vi "Results Analyser.vi"() -> ()   [LabVIEW 2020]
panel:
  in  "Reset":bool
  out "Total Files":u32
  in  "Calculate":bool
  in  "Quit":bool
  in  "Lower Limit":string
  in  "Upper Limit":string
  out "Analysis":T1={"Target"=4.0, "Average"=4.07375, "Standard Deviation"=0.10336309095334055, "Cp"=3.2248777610937, "Cpu"=2.9870430262130383, "Cpl"=3.462712495974362, "Cpk"=2.9870430262130383}
  out "Results":dbl[](array[numeric])=[4.0, 4.1, 4.07, 4.1, 4.0, 4.05, 4.3, 3.97]
  out "Graph":picture
  out "Histogram":picture
  in  "Tests":i32(listbox)
  out "Test List":string[](array[string])
  out "Files":path[](array[path])
  in  "Add Files":bool
  in  "Aborted":bool
  in  "Fail":bool
  in  "Pass":bool=TRUE
  in  "Results Directory":path=path "C:/Results/test"
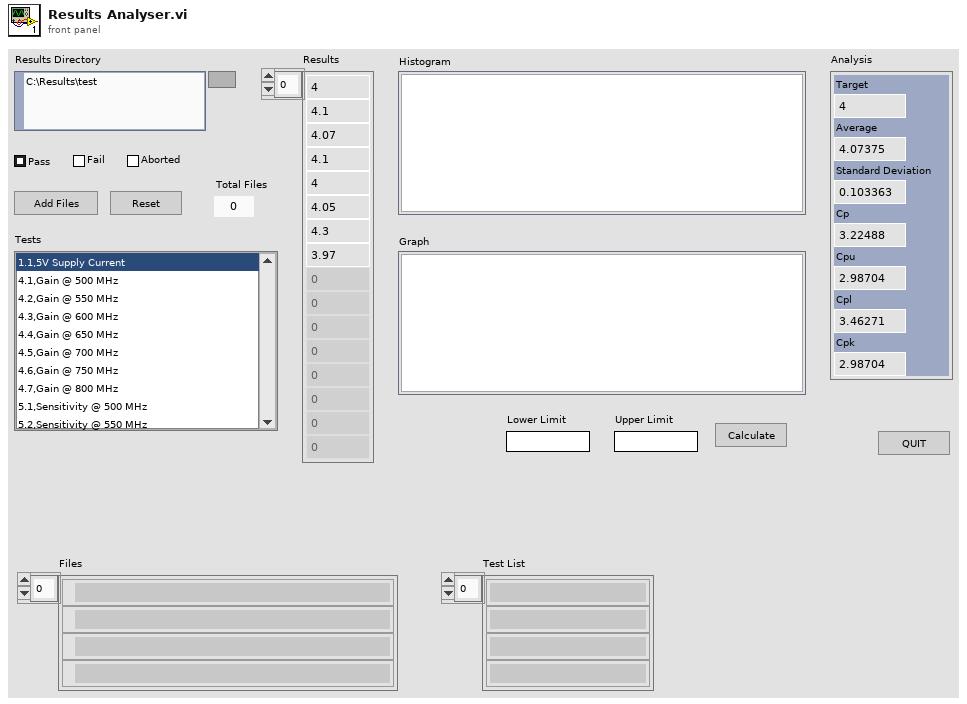
[diagram p1: front panel]
types:
  T1 = cluster{"Target":dbl, "Average":dbl, "Standard Deviation":dbl, "Cp":dbl, "Cpu":dbl, "Cpl":dbl, "Cpk":dbl}
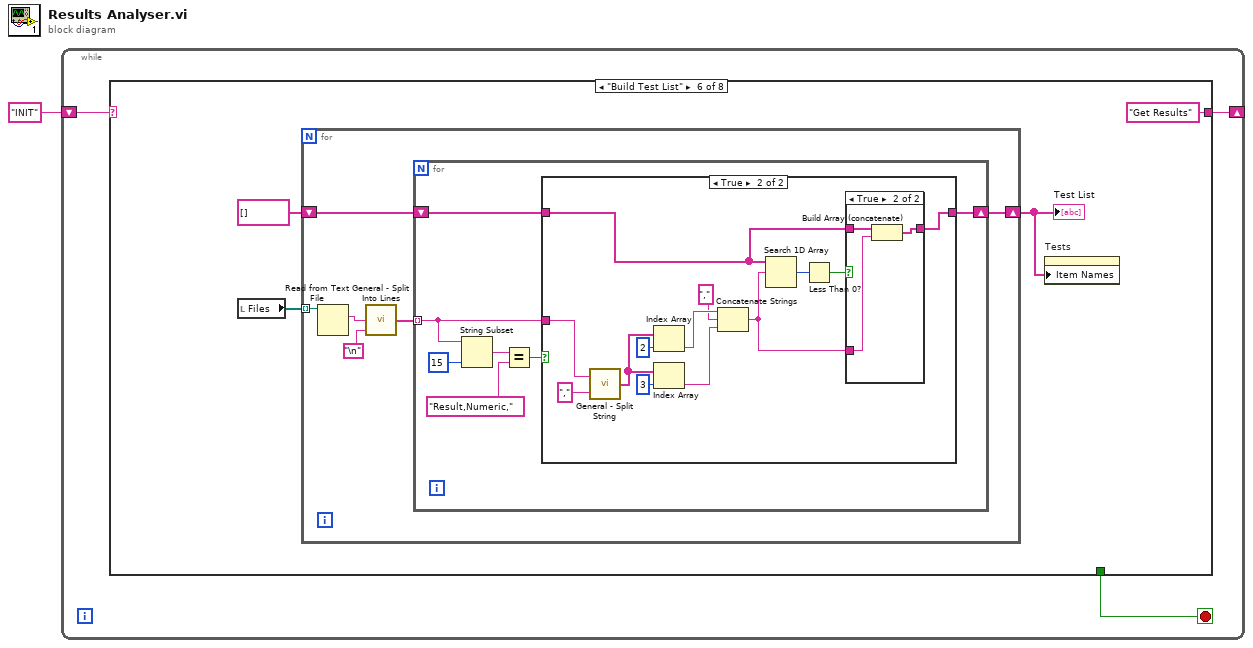
[diagram p0: block diagram]
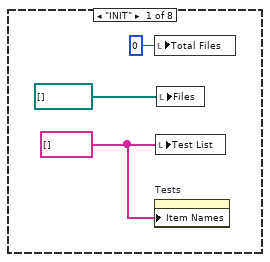
[diagram p2: hidden frame]
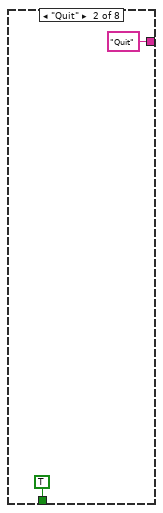
[diagram p3: hidden frame]
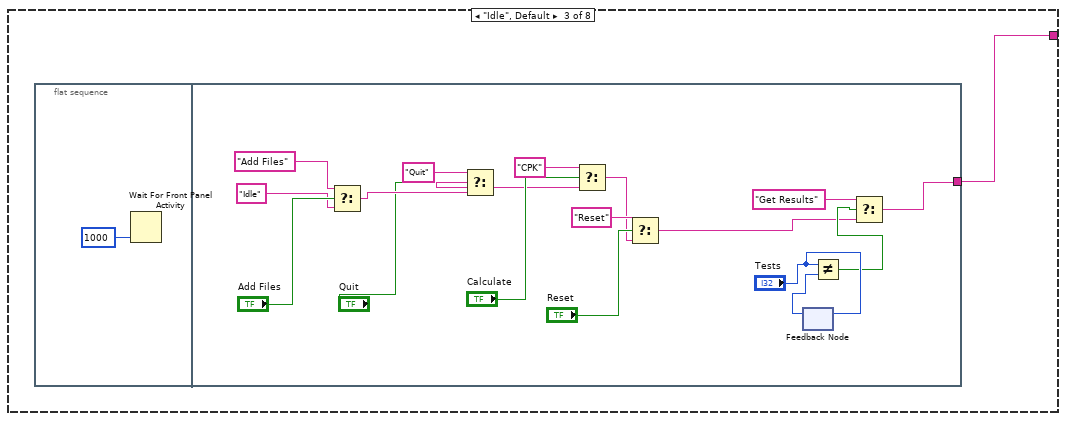
[diagram p4: hidden frame]
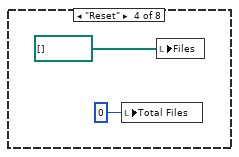
[diagram p5: hidden frame]
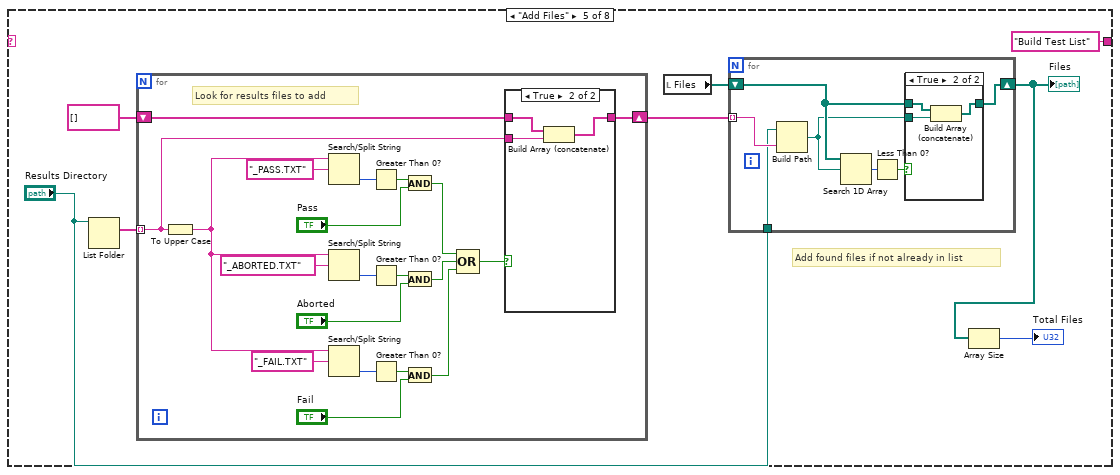
[diagram p6: hidden frame]
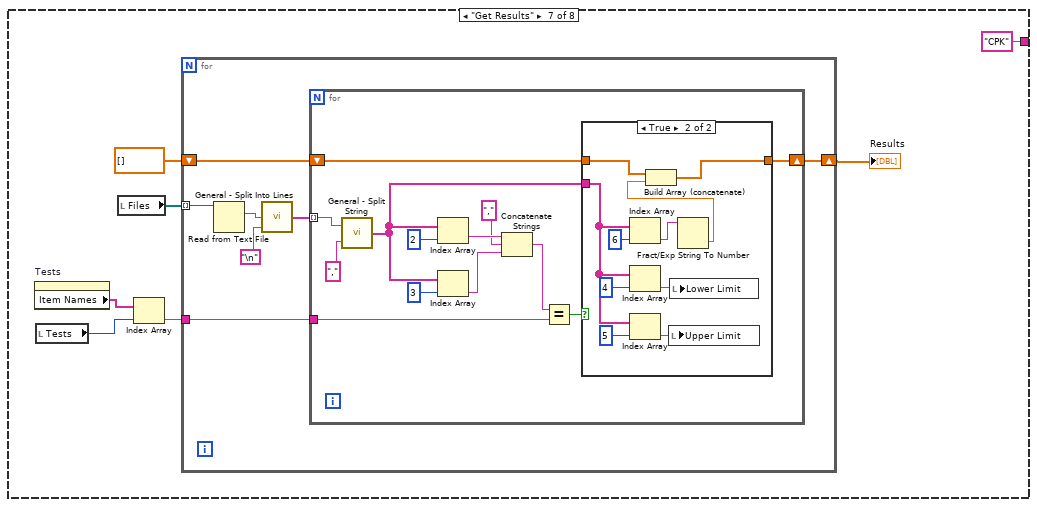
[diagram p11: hidden frame]
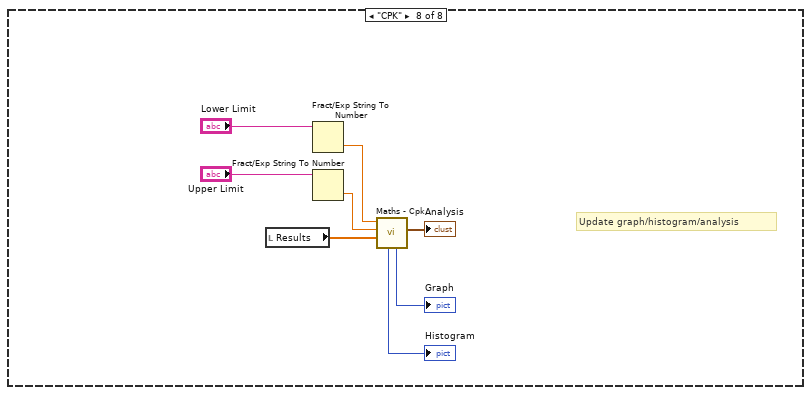
[diagram p13: hidden frame]
diagram:
  n1 = while {
    shift-right: [w3] -> _
    shift-left: "INIT" -> [w4]
    stop <- w2 stop-if-true
    n2 = case shown="\"Build Test List\"" w4 {
      tunnel: [_ "Quit" w10 _ "Build Test List" "Get Results" "CPK" _] -> w3
      tunnel: [_ TRUE _ _ _ _ _ _] -> w2
      frame "INIT" {
        w5 = string[] []
        n3 = local write "Total Files"(u32 0 ("Total Files")) -> ()
        n4 = property on="Tests" class="LstBox (strict)"("Item Names"=w5) -> ()  [unwired: 2 in, 2 out]
        n5 = local write "Test List"(w5) -> ()
        n6 = local write "Files"(path[] []) -> ()
      }
      frame "Quit" {
      }
      frame "Idle", Default {
        n7 = flat-sequence {
          tunnel: [w20] -> w10
          frame #0 {
            n8 = Wait For Front Panel Activity(1:1000 ("timeout ms (-1 never timeout)")) -> ()  [unwired: 2 in, 1 out]
          }
          frame #1 {
            n9 = Select(t="Add Files", s="Add Files", f="Idle") -> (s? t:f=w25:string)
            n10 = Select(t="Quit", s="Quit", f=w25) -> (s? t:f=w24:string)
            n11 = Select(t="CPK", s="Calculate", f=w24) -> (s? t:f=w13:string)
            n12 = Select(t="Reset", s="Reset", f=w13) -> (s? t:f=w12:string)
            n13 = feedback-in #1("Tests") -> ()
            n14 = feedback #1() -> (w18:i32)  [unwired: 1 in]
            n15 = Not Equal?(x="Tests", y=w18) -> (x != y?=w16:bool)
            n16 = Select(t="Get Results", s=w16, f=w12) -> (s? t:f=w20:string)
          }
        }
      }
      frame "Reset" {
        n17 = local write "Total Files"(u32 0 ("Total Files")) -> ()
        n18 = local write "Files"(path[] []) -> ()
      }
      frame "Add Files" {
        # "Add found files if not already in list"
        n19 = List Folder(path="Results Directory") -> (filenames=w39:string[])  [unwired: 3 in, 3 out]
        n20 = for {
          tunnel: w39 -> [w51] mode=indexing
          shift-right: [w53] -> w37
          shift-left: string[] [] -> [w54]
          # "Look for results files to add"
          n21 = To Upper Case(1:w51) -> (0:w52:string)
          n22 = Search/Split String(string=w52, search string/char (-)="_PASS.TXT") -> (offset of match=w64:i32)  [unwired: 1 in, 2 out]
          n23 = Search/Split String(string=w52, search string/char (-)="_ABORTED.TXT") -> (offset of match=w63:i32)  [unwired: 1 in, 2 out]
          n24 = Search/Split String(string=w52, search string/char (-)="_FAIL.TXT") -> (offset of match=w62:i32)  [unwired: 1 in, 2 out]
          n25 = Greater Than 0?(x=w64) -> (x > 0?=w61:bool)
          n26 = Greater Than 0?(x=w63) -> (x > 0?=w60:bool)
          n27 = Greater Than 0?(x=w62) -> (x > 0?=w59:bool)
          n28 = And(x=w61, y="Pass") -> (x .and. y?=w67:bool)
          n29 = And(x=w60, y="Aborted") -> (x .and. y?=w66:bool)
          n30 = And(x=w59, y="Fail") -> (x .and. y?=w65:bool)
          n31 = Compound Arithmetic op=OR(w67, w66, w65) -> (w55:bool)
          n32 = case shown="True" w55 {
            tunnel: w54 -> [w71 w73]
            tunnel: [w71 w74] -> w53
            tunnel: w51 -> [_ w72]
            frame False {
            }
            frame True {
              n33 = Build Array (concatenate)(w73, w72) -> (w74:string[])
            }
          }
        }
        n34 = local read "Files"() -> (w33:path[])
        n35 = for {
          tunnel: w37 -> [w46] mode=indexing
          tunnel: "Results Directory" -> [w45]
          shift-right: [w40] -> w32
          shift-left: w33 -> [w42]
          n36 = Build Path(base path=w45, name or relative path=w46) -> (appended path=w41:path)
          n37 = Search 1D Array(1D array=w42, element=w41) -> (index of element=w44:i32)  [unwired: 1 in]
          n38 = Less Than 0?(x=w44) -> (x < 0?=w43:bool)
          n39 = case shown="True" w43 {
            tunnel: w42 -> [w47 w50]
            tunnel: [w47 w49] -> w40
            tunnel: w41 -> [_ w48]
            frame False {
            }
            frame True {
              n40 = Build Array (concatenate)(w50, w48) -> (w49:path[])
            }
          }
        }
        "Files" <- w32
        n41 = Array Size(array=w32) -> (size(s)=→"Total Files":i32)
      }
      frame "Build Test List" {
        n42 = local read "Files"() -> (w78:path[])
        n43 = for {
          tunnel: w78 -> [w84] mode=indexing
          shift-right: [w79] -> w76
          shift-left: string[] [] -> [w80]
          n44 = Read from Text File(file (use dialog)=w84) -> (text=w83:string)  [unwired: 3 in, 3 out]
          n45 = call "General - Split Into Lines.vi"("Line Termination Character"="\n", "String"=w83) -> ("Array"=w81:string[])  [unwired: 3 in]
          n46 = for {
            tunnel: w81 -> [w87] mode=indexing
            shift-right: [w85] -> w79
            shift-left: w80 -> [w86]
            n47 = String Subset(string=w87, length (rest)=15 ("length (rest)")) -> (substring=w90:string)  [unwired: 1 in]
            n48 = Equal?(x=w90, y="Result,Numeric,") -> (x = y?=w88:bool)
            n49 = case shown="True" w88 {
              tunnel: w87 -> [_ w105]
              tunnel: w86 -> [w92 w95]
              tunnel: [w92 w94] -> w85
              frame False {
              }
              frame True {
                n50 = call "General - Split String.vi"("Delimeter (;)"=",", "String"=w105) -> ("String Array"=w103:string[])
                n51 = Index Array(array=w103, index=2) -> (element=w100:string)
                n52 = Index Array(array=w103, index=3) -> (element=w99:string)
                n53 = Concatenate Strings(w100, ",", w99) -> (w93:string)
                n54 = Search 1D Array(1D array=w95, element=w93) -> (index of element=w97:i32)  [unwired: 1 in]
                n55 = Less Than 0?(x=w97) -> (x < 0?=w96:bool)
                n56 = case shown="True" w96 {
                  tunnel: w95 -> [w106 w109]
                  tunnel: [w106 w108] -> w94
                  tunnel: w93 -> [_ w107]
                  frame False {
                  }
                  frame True {
                    n57 = Build Array (concatenate)(w109, w107) -> (w108:string[])
                  }
                }
              }
            }
          }
        }
        "Test List" <- w76
        n58 = property on="Tests" class="LstBox (strict)"("Item Names"=w76) -> ()  [unwired: 2 in, 2 out]
      }
      frame "Get Results" {
        n59 = property on="Tests" class="LstBox (strict)"() -> ("Item Names"=w116:string[])  [unwired: 2 in, 2 out]
        n60 = local read "Tests"() -> (w115:i32)
        n61 = local read "Files"() -> (w113:path[])
        n62 = Index Array(array=w116, index=w115) -> (element=w114:string)
        n63 = for {
          tunnel: w114 -> [w119]
          tunnel: w113 -> [w123] mode=indexing
          shift-right: [w117] -> w112
          shift-left: dbl[] [] -> [w118]
          n64 = Read from Text File(file (use dialog)=w123) -> (text=w122:string)  [unwired: 3 in, 3 out]
          n65 = call "General - Split Into Lines.vi"("Line Termination Character"="\n", "String"=w122) -> ("Array"=w120:string[])  [unwired: 3 in]
          n66 = for {
            tunnel: w120 -> [w136] mode=indexing
            tunnel: w119 -> [w128]
            shift-right: [w126] -> w117
            shift-left: w118 -> [w127]
            n67 = call "General - Split String.vi"("Delimeter (;)"=",", "String"=w136) -> ("String Array"=w125:string[])
            n68 = Index Array(array=w125, index=2) -> (element=w132:string)
            n69 = Index Array(array=w125, index=3) -> (element=w131:string)
            n70 = Concatenate Strings(w132, ",", w131) -> (w129:string)
            n71 = Equal?(x=w129, y=w128) -> (x = y?=w124:bool)
            n72 = case shown="True" w124 {
              tunnel: w127 -> [w137 w147]
              tunnel: [w137 w146] -> w126
              tunnel: w125 -> [_ w142]
              frame False {
              }
              frame True {
                n73 = Index Array(array=w142, index=6) -> (element=w144:string)
                n74 = Index Array(array=w142, index=4) -> (element=w139:string)
                n75 = Index Array(array=w142, index=5) -> (element=w138:string)
                n76 = local write "Upper Limit"(w138) -> ()
                n77 = local write "Lower Limit"(w139) -> ()
                n78 = Fract/Exp String To Number(string=w144) -> (number=w143:dbl)  [unwired: 3 in, 1 out]
                n79 = Build Array (concatenate)(w147, w143) -> (w146:dbl[])
              }
            }
          }
        }
        "Results" <- w112
      }
      frame "CPK" {
        # "Update graph/histogram/analysis"
        n80 = local read "Results"() -> (w155:dbl[])
        n81 = Fract/Exp String To Number(string="Lower Limit") -> (number=w152:dbl)  [unwired: 3 in, 1 out]
        n82 = Fract/Exp String To Number(string="Upper Limit") -> (number=w151:dbl)  [unwired: 3 in, 1 out]
        n83 = call "Maths - Cpk.vi"("Results"=w155, "Upper Limit"=w151, "Lower Limit"=w152) -> ("Results"=→"Analysis":T1, "Graph"=→"Graph":picture, "Histogram"=→"Histogram":picture)  [unwired: 6 in]
      }
    }
  }
